vi "Day 17.vi"() -> ()   [LabVIEW 2021]
panel:
  in  "Input File":enum32{"example input", "input"}(radio)
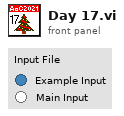
[diagram p1: front panel]
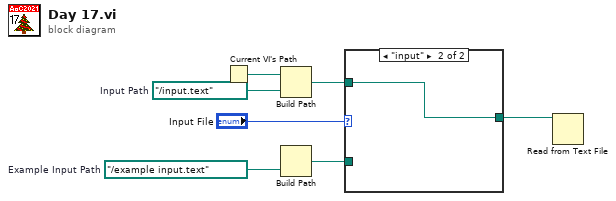
[diagram p0: block diagram]
diagram:
  w5 = path "../example input.text"  # Example Input Path
  w7 = path "../input.text"  # Input Path
  n1 = Current VI's Path() -> (path=w6:path)
  n2 = Build Path(base path=w6, name or relative path=w7) -> (appended path=w3:path)
  n3 = Build Path(name or relative path=w5) -> (appended path=w2:path)  [unwired: 1 in]
  n4 = case shown="\"input\"" "Input File" {
    tunnel: w3 -> [_ w9]
    tunnel: w2 -> [w8 _]
    tunnel: [w8 w9] -> w1
    frame "example input" {
    }
    frame "input" {
    }
  }
  n5 = Read from Text File(file (use dialog)=w1) -> ()  [unwired: 3 in, 4 out]
